vi "handleRejectedCommand.vi"(8 "error in (no error)":errorcluster, 10 "CommandValue":T1, 11 "Model in":refnum<class "Model.lvclass">) -> (0 "error out":errorcluster, 3 "Model out":refnum<class "Model.lvclass">)   [LabVIEW 2016, in "Model.lvclass"]
uses:
  Model.lvclass
  Typedefs/CommandValue.ctl
  Typedefs/RejectedCommand.ctl
  Typedefs/StateValue.ctl
  Typedefs/PubDataSV.ctl
  Model.lvclass/Model.ctl
  PubSubDataEvent/PubSubDataEvent.lvclass/PubSubDataEvent.ctl
  PubSubDataEvent/Read pubDataEvents.vi
  Typedefs/EXATypedefs.lvlib
panel:
  # "w"
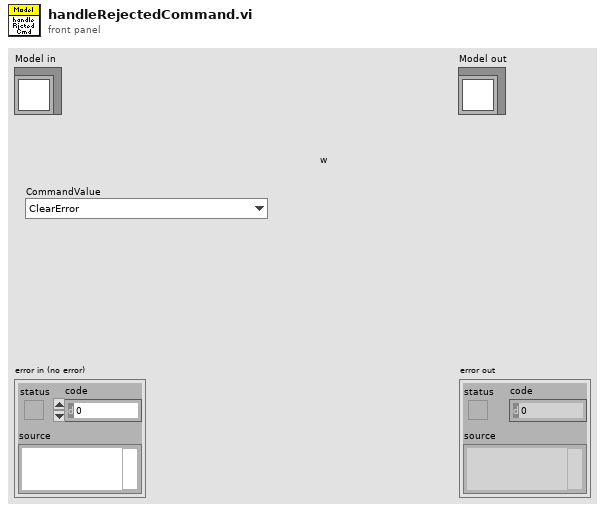
[diagram p1: front panel]
types:
  T1 = typedef "EXATypedefs.lvlib/CommandValue.ctl" = enum16{"ClearError", "Disable", "Enable", "Exit", "GoToStandby", "OnHeartbeat", "OnIncomingMessagingError", "OnInterrupt", "Start"}
  T2 = typedef "EXATypedefs.lvlib/PubDataSV.ctl" = enum16{"DetailedState", "ErrorCode", "Heartbeat", "LoopTime_ms", "LoopTimeOutOfRange", "RejectedCommand", "SummaryState", "Timestamp"}
  T3 = typedef "EXATypedefs.lvlib/RejectedCommand.ctl" = cluster{"CommandValue":T1, "StateValue":T4, "Time Stamp":dbl}
  T4 = typedef "EXATypedefs.lvlib/StateValue.ctl" = enum16{"DisabledState", "EnabledState", "FaultState", "OffState", "StandbyState"}
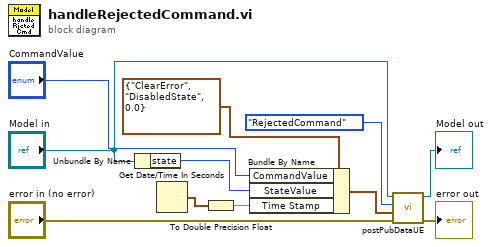
[diagram p0: block diagram]
diagram:
  n1 = Unbundle By Name("Model in") -> ("state"=w9:T4)
  n2 = Get Date/Time In Seconds() -> (seconds since 1Jan1904=w1:timestamp)
  n3 = To Double Precision Float(number=w1) -> (double precision float=w2:dbl)
  n4 = Bundle By Name(cluster=T3 {"CommandValue"=enum."ClearError", "StateValue"=enum."DisabledState", "Time Stamp"=0.0} ("RejectedCommandSV"), "CommandValue"="CommandValue", "StateValue"=w9, "Time Stamp"=w2) -> (w5:T3)
  n5 = call "postPubDataUE.vi"("error in (no error)"="error in (no error)", "value"=w5, "pubDataSV"=PubDataSV."RejectedCommand", "Model in"="Model in") -> ("error out"=→"error out":errorcluster, "Model out"=→"Model out":refnum<class "Model.lvclass">)  [unwired: 6 in]
